vi "Write grapher output.vi"(0 "Data output file":path, 5 "Time":i64, 7 "Polarization":dbl, 9 "Frequency":dbl, 11 "Rate":dbl) -> ()   [LabVIEW 2015]
uses:
  <vilib>/Utility/file.llb/Write Delimited Spreadsheet (string).vi
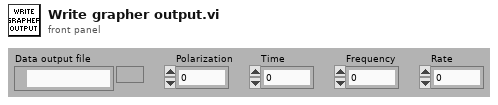
[diagram p1: front panel]
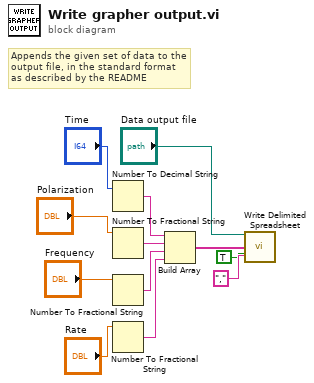
[diagram p0: block diagram]
diagram:
  # "Appends the given set of data to the\noutput file, in the standard format\nas described by the README"
  n1 = Number To Decimal String(number="Time") -> (decimal integer string=w7:string)  [unwired: 1 in]
  n2 = Number To Fractional String(number="Polarization") -> (F-format string=w8:string)  [unwired: 3 in]
  n3 = Number To Fractional String(number="Frequency") -> (F-format string=w9:string)  [unwired: 3 in]
  n4 = Number To Fractional String(number="Rate") -> (F-format string=w10:string)  [unwired: 3 in]
  n5 = Build Array(w7, w8, w9, w10) -> (w2:string[])
  n6 = call-poly <vilib>:"Write Delimited Spreadsheet.vi"("file path (dialog if empty)"="Data output file", "1D data"=w2, "append to file? (F)"=TRUE ("append to file? (new file:F)"), "delimiter (\\t)"="," ("delimiter (\\t)")) -> ()  [unwired: 10 in, 2 out]
